vi "SLSC Switch - Initialize with Topology (Reservation Group and Override Switches).vi"(6 "reservation group":string, 7 "switches json":string, 8 "error in (no error)":errorcluster, 9 "reset device":bool=TRUE, 10 "topology":string, 11 "device":refnum<k21>) -> (0 "error out":errorcluster, 3 "session out":T1)   [LabVIEW 2017, in "NI-SWITCH Messaging.lvlib" / "NI-SWITCH Consumer.lvclass"]
doc: "Returns a session handle used to identify the SLSC Switch module in all subsequent driver calls and sets the topology of the switch module."
uses:
  NI-SWITCH Consumer.lvclass
  <vilib>/userdefined/High Color/SLSC_Switch/nislscslSession.ctl
panel:
  in  "session in":T1
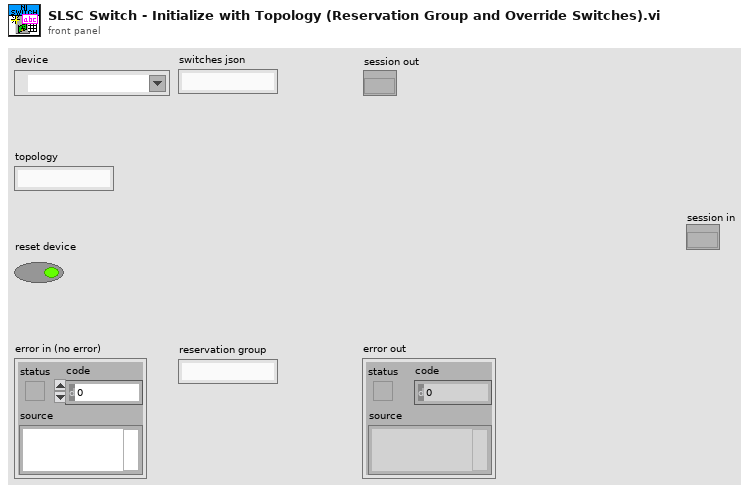
[diagram p1: front panel]
types:
  T1 = typedef "nislscslSession.ctl" = refnum<k20>
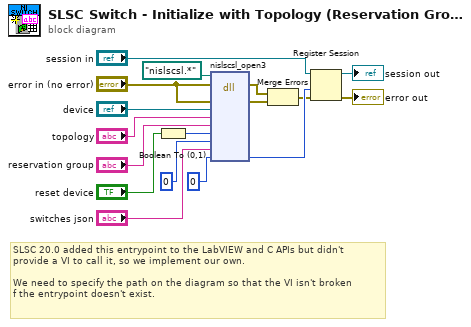
[diagram p0: block diagram]
diagram:
  # "SLSC 20.0 added this entrypoint to the LabVIEW and C APIs but didn't\nprovide a VI to call it, so we implement our own.\n\nWe need to specify the path on the diagram so that the VI isn't broken \nf the entrypoint doesn't exist."
  n1 = Boolean To (0,1)(Boolean="reset device") -> (0, 1=w6:i16)
  n2 = dll-call lib="nislscsl.*" fn="nislscsl_open3"(path in=path "nislscsl.*", error in="error in (no error)", "errorCluster"="error in (no error)", "deviceIdentifier"="device", "topologyName"="topology", "reservationGroup"="reservation group", "reset"=w6, "simulate"=u8 0, "capabilities"="switches json", "sessionHandlePtr"=u64 0) -> (error out=w14:errorcluster, "errorCluster"=w13:errorcluster, "sessionHandlePtr"=w12:u64)  [unwired: 8 in, 1 out]
  n3 = Merge Errors(w14, w13) -> (w11:errorcluster)
  n4 = Register Session(8:w11, 9:w12, 11:"session in") -> (0:→"error out":errorcluster, 3:→"session out":T1)  [unwired: 2 in]
